vi "UTL_PopulateStatusCtrls.vi"(8 "error in (no error)":errorcluster, 9 "Status":u32, 10 "Recipe":string, 11 "ComNum":i32) -> (0 "error out":errorcluster, 3 "output cluster":T1)   [LabVIEW 2024]
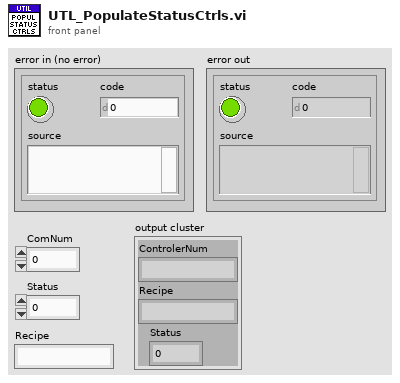
[diagram p1: front panel]
types:
  T1 = cluster{"ControlerNum":string, "Recipe":string, "Status":u32}
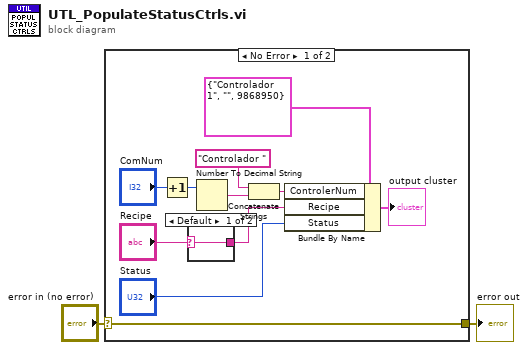
[diagram p0: block diagram]
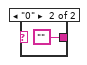
[diagram p2: hidden frame]
diagram:
  n1 = case shown="No Error" "error in (no error)" {
    selector: "error in (no error)" -> [w13 w16]
    tunnel: [w13 w16] -> w1
    frame No Error {
      n2 = Increment(x="ComNum") -> (x+1=w10:i32)
      n3 = case shown="Default" "Recipe" {
        selector: "Recipe" -> [w14 _]
        tunnel: [w14 ""] -> w3
        frame Default {
        }
        frame "0" {
        }
      }
      n4 = Number To Decimal String(number=w10) -> (decimal integer string=w12:string)  [unwired: 1 in]
      n5 = Concatenate Strings("Controlador " ("Control#"), w12) -> (w7:string)
      n6 = Bundle By Name(cluster=T1 {"ControlerNum"="Controlador 1", "Recipe"="", "Status"=9868950} ("Controllers Load"), "ControlerNum"=w7, "Recipe"=w3, "Status"="Status") -> (→"output cluster":T1)
    }
    frame Error {
    }
  }
  "error out" <- w1
